vi "Control - Diesel - Cranking.vi"(0 "Control Inputs":T4={"Engine Speed [RPM]"=0.0, "Engine Status"=enum."STALLED", "Load Control \nMode"=enum."High-Idle Governor", "dt(s)"=0.0, "Number of Cylinders"=0, "Engine Displacement [cc]"=0.0, "StoichAFR"=0.0, "Q.LHV Fuel [kJ/kg]"=0.0, "BattV PSU [V]"=0.0, "12V PSU [V]"=0.0, "5V PSU [V]"=0.0, "Pedal Position [%]"=0.0, "Oil Pressure [kPa]"=0.0, "Oil Temp [C]"=0.0, "Oil Level [%]"=0.0, "Engine Coolant Temp (ECT) [C]"=0.0, "Engine Coolant Pressure [kPa]"=0.0, "Rail Pressure [bar]"=0.0, "Fuel Pressure [kPa]"=0.0, "Fuel Temp [C]"=0.0, "Vacuum Pressure [kPa]"=0.0, "Throttle Position [%]"=0.0, "Cam1 Advance [CAD]"=0.0, "Cam2 Advance [CAD]"=0.0, "Cam3 Advance [CAD]"=0.0, "Cam4 Advance [CAD]"=0.0, "CA50 Control Output [CAD]"=[], "CA50 Control Output Valid"=[], "Intake Air Temp (IAT) [C]"=0.0, "Barometric Air Pressure [kPa]"=0.0, "Intake Air Rel. Humidity [%]"=0.0, "Mass Air Flow (MAF) [kg/hr]"=0.0, "Turbo Inlet Air Pressure [kPa]"=0.0, "Turbo Inlet Air Temp [C]"=0.0, "Turbo Outlet Air Pressure [kPa]"=0.0, "Turbo Outlet Air Temp [C]"=0.0, "CAC Outlet Pressure [kPa]"=0.0, "CAC Outlet Temp [C]"=0.0, "Intake Manifold Pressure (MAP) [kPa]"=0.0, "Intake Manifold Temp (MAT) [C]"=0.0, "Exhaust Manifold Pressure [kPa]"=0.0, "Exhaust Manifold Temp [C]"=0.0, "HighP EGR Cooler Outlet Pressure [kPa]"=0.0, "HighP EGR Cooler Outlet Temp [C]"=0.0, "HighP EGR Differential Pressure [kPa]"=0.0, "HighP EGR Valve Position [%]"=0.0, "Turbo Outlet Exhaust Pressure [kPa]"=0.0, "Turbo Outlet Exhaust Temp [C]"=0.0, "VGT Position 1 [%]"=0.0, "VGT Position 2 [%]"=0.0, "Turbo Speed 1 [RPM]"=0.0, "Turbo Speed 2 [RPM]"=0.0, "LowP EGR Differential Pressure [kPa]"=0.0, "LowP EGR Valve Position [%]"=0.0, "UEGO1Lambda"=0.0, "UEGO1_Hot"=FALSE, "UEGO2Lambda"=0.0, "UEGO2_Hot"=FALSE, "Knock Intensity"=[], "Knock"=[]} {"Knock Intensity" format="%.2f"; "CA50 Control Output [CAD]" format="%.2f"; "Exhaust Manifold Temp [C]" format="%#_6f"; "UEGO2Lambda" format="%.2f"; "Intake Manifold Temp (MAT) [C]" format="%#_6f"; "UEGO1Lambda" format="%.2f"}, 1 "Available Air Mass [mg/cyc]":sgl, 5 "Control Outputs In":T1) -> (19 "Control Outputs":T1)   [LabVIEW 2015, in "ECS-RT.lvlib"]
uses:
  ECS-RT.lvlib
  Typedefs/Control Inputs/Control Inputs.ctl
  Typedefs/EPT/Engine Status.ctl
  Typedefs/MISC/Load Control Mode.ctl
  Typedefs/Control Outputs/Control Outputs.ctl
  Typedefs/Control Outputs/Injection Quantity.ctl
  Typedefs/Control Outputs/Injection Timing.ctl
  ECS-Shared.lvlib
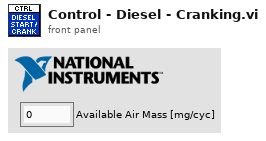
[diagram p1: front panel]
types:
  T1 = typedef "ECS-Shared.lvlib/Control Outputs.ctl" = cluster{"Pedal Desired [%]":sgl, "MEP Desired [bar]":sgl, "Fuel Desired [mg/cyc]":sgl, "Intake MAP Desired [kPa]":sgl, "Cam1 Advance Setpoint [CAD]":sgl, "Cam2 Advance Setpoint [CAD]":sgl, "HighP EGR Position Setpoint [%Open]":sgl, "LowP EGR Position Setpoint [%Open]":sgl, "Rail Pressure Setpoint [bar]":sgl, "Wastegate1 Position Setpoint [%Open]":sgl, "Wastegate2 Position Setpoint [%Open]":sgl, "VGT1 Position Setpoint [%Open]":sgl, "VGT2 Position Setpoint [%Open]":sgl, "Throttle1 Position Setpoint [%Open]":sgl, "Throttle2 Position Setpoint [%Open]":sgl, "TurboBPV Position Setpoint [%Open]":sgl, "Spark Dwells [msec]":sgl[], "Spark Timings [DBTDC]":sgl[], "PFI Quantities [mg/inj]":sgl[], "PFI Timings [DBTDC]":sgl[], "DI Quantities [mg/inj]":T2[], "DI Timings [DBTDC]":T3[]}
  T2 = typedef "ECS-Shared.lvlib/Injection Quantity.ctl" = cluster{"Pilot1Quantity [mg/inj]":sgl, "Pilot2Quantity [mg/inj]":sgl, "MainQuantity [mg/inj]":sgl, "Post1Quantity [mg/inj]":sgl, "Post2Quantity [mg/inj]":sgl}
  T3 = typedef "ECS-Shared.lvlib/Injection Timing.ctl" = cluster{"Pilot1SOI [DBTDC]":sgl, "Pilot2SOI [DBTDC]":sgl, "MainSOI [DBTDC]":sgl, "Post1SOI [DBTDC]":sgl, "Post2SOI [DBTDC]":sgl}
  T4 = typedef "ECS-Shared.lvlib/Control Inputs.ctl" = cluster{"Engine Speed [RPM]":sgl, "Engine Status":T5, "Load Control \nMode":T6, "dt(s)":sgl, "Number of Cylinders":u8, "Engine Displacement [cc]":sgl, "StoichAFR":sgl, "Q.LHV Fuel [kJ/kg]":sgl, "BattV PSU [V]":sgl, "12V PSU [V]":sgl, "5V PSU [V]":sgl, "Pedal Position [%]":sgl, "Oil Pressure [kPa]":sgl, "Oil Temp [C]":sgl, "Oil Level [%]":sgl, "Engine Coolant Temp (ECT) [C]":sgl, "Engine Coolant Pressure [kPa]":sgl, "Rail Pressure [bar]":sgl, "Fuel Pressure [kPa]":sgl, "Fuel Temp [C]":sgl, "Vacuum Pressure [kPa]":sgl, "Throttle Position [%]":sgl, "Cam1 Advance [CAD]":sgl, "Cam2 Advance [CAD]":sgl, "Cam3 Advance [CAD]":sgl, "Cam4 Advance [CAD]":sgl, "CA50 Control Output [CAD]":sgl[], "CA50 Control Output Valid":bool[], "Intake Air Temp (IAT) [C]":sgl, "Barometric Air Pressure [kPa]":sgl, "Intake Air Rel. Humidity [%]":sgl, "Mass Air Flow (MAF) [kg/hr]":sgl, "Turbo Inlet Air Pressure [kPa]":sgl, "Turbo Inlet Air Temp [C]":sgl, "Turbo Outlet Air Pressure [kPa]":sgl, "Turbo Outlet Air Temp [C]":sgl, "CAC Outlet Pressure [kPa]":sgl, "CAC Outlet Temp [C]":sgl, "Intake Manifold Pressure (MAP) [kPa]":sgl, "Intake Manifold Temp (MAT) [C]":sgl, "Exhaust Manifold Pressure [kPa]":sgl, "Exhaust Manifold Temp [C]":sgl, "HighP EGR Cooler Outlet Pressure [kPa]":sgl, "HighP EGR Cooler Outlet Temp [C]":sgl, "HighP EGR Differential Pressure [kPa]":sgl, "HighP EGR Valve Position [%]":sgl, "Turbo Outlet Exhaust Pressure [kPa]":sgl, "Turbo Outlet Exhaust Temp [C]":sgl, "VGT Position 1 [%]":sgl, "VGT Position 2 [%]":sgl, "Turbo Speed 1 [RPM]":sgl, "Turbo Speed 2 [RPM]":sgl, "LowP EGR Differential Pressure [kPa]":sgl, "LowP EGR Valve Position [%]":sgl, "UEGO1Lambda":sgl, "UEGO1_Hot":bool, "UEGO2Lambda":sgl, "UEGO2_Hot":bool, "Knock Intensity":sgl[], "Knock":bool[]}
  T5 = typedef "ECS-Shared.lvlib/Engine Status.ctl" = enum16{"OFF", "STALLED", "CRANKING", "RUNNING", "ACCEL", "DECEL", "SAFE"}
  T6 = typedef "ECS-Shared.lvlib/Load Control Mode.ctl" = enum16{"No Governor", "Low-Idle Governor", "High-Idle Governor"}
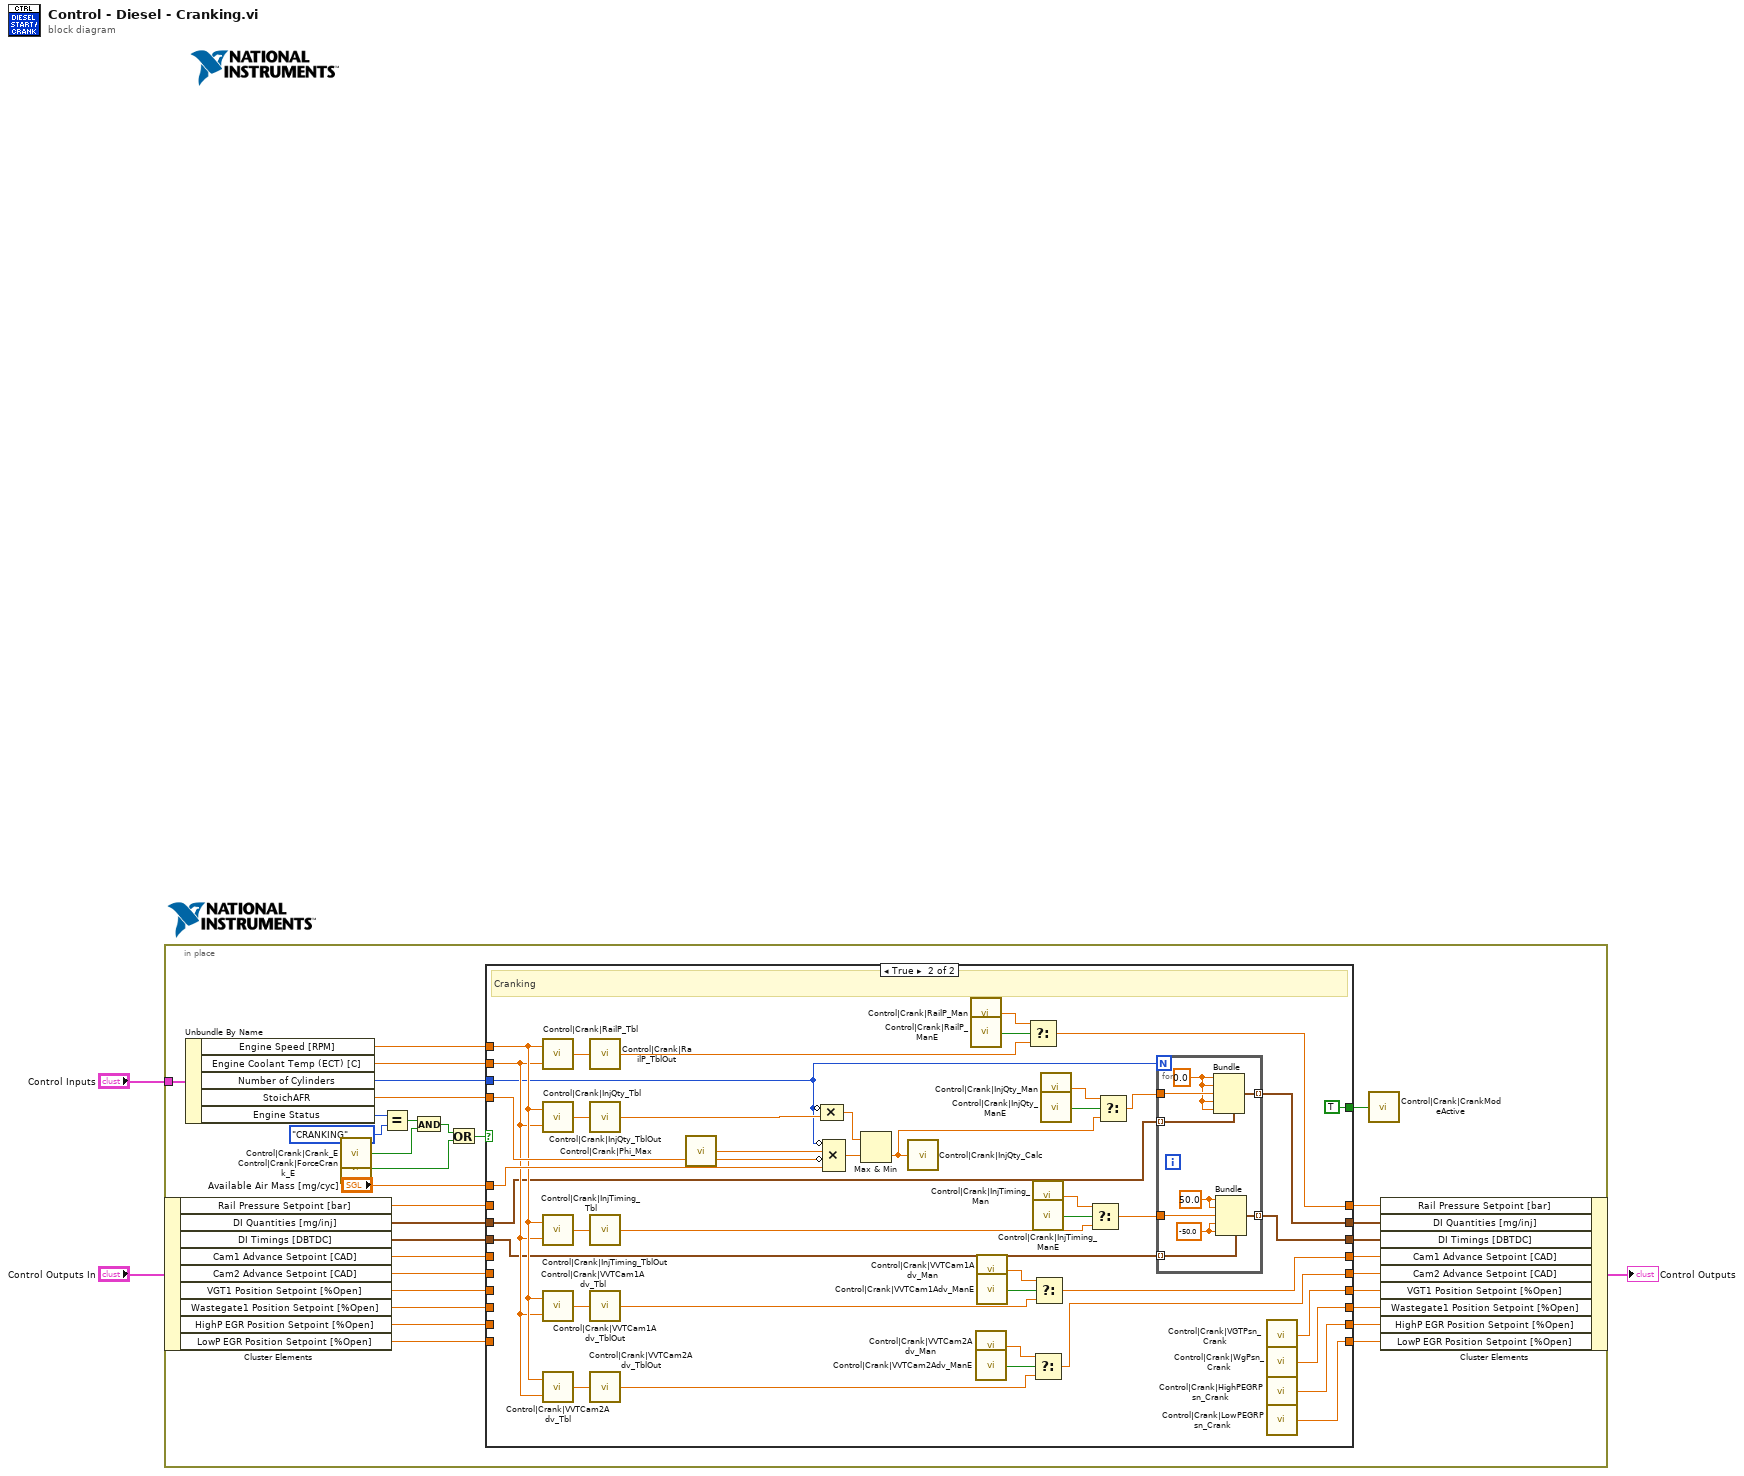
[diagram p0: block diagram]
diagram:
  n1 = in-place {
    in-place-border: "Control Inputs" -> [w31]
    n2 = in-place-cluster #1("Control Outputs In") -> ("Rail Pressure Setpoint [bar]"=w21:sgl, "DI Quantities [mg/inj]"=w20:T2[], "DI Timings [DBTDC]"=w19:T3[], "Cam1 Advance Setpoint [CAD]"=w18:sgl, "Cam2 Advance Setpoint [CAD]"=w17:sgl, "VGT1 Position Setpoint [%Open]"=w16:sgl, "Wastegate1 Position Setpoint [%Open]"=w15:sgl, "HighP EGR Position Setpoint [%Open]"=w14:sgl, "LowP EGR Position Setpoint [%Open]"=w13:sgl)
    n3 = Unbundle By Name(w31) -> ("Engine Speed [RPM]"=w35:sgl, "Engine Coolant Temp (ECT) [C]"=w34:sgl, "Number of Cylinders"=w33:u8, "StoichAFR"=w32:sgl, "Engine Status"=w29:T5)
    n4 = call "Control|Crank|Crank_E"() -> ("Value"=w26:bool)
    n5 = call "Control|Crank|ForceCrank_E"() -> ("Value"=w24:bool)
    n6 = Equal?(x=w29, y=Engine_Status."CRANKING" ("Engine Status")) -> (x = y?=w27:bool)
    n7 = And(x=w27, y=w26) -> (x .and. y?=w23:bool)
    n8 = Or(x=w23, y=w24) -> (x .or. y?=w25:bool)
    n9 = case shown="True" w25 {
      tunnel: w35 -> [_ w59]
      tunnel: w34 -> [_ w58]
      tunnel: w33 -> [_ w45]
      tunnel: w32 -> [_ w73]
      tunnel: "Available Air Mass [mg/cyc]" -> [_ w72]
      tunnel: [_ TRUE] -> w30
      tunnel: w21 -> [w36 _]
      tunnel: w20 -> [w37 w51]
      tunnel: w19 -> [w38 w46]
      tunnel: w18 -> [w39 _]
      tunnel: w17 -> [w40 _]
      tunnel: w16 -> [w41 _]
      tunnel: w15 -> [w42 _]
      tunnel: w14 -> [w43 _]
      tunnel: w13 -> [w44 _]
      tunnel: [w44 w52] -> w12
      tunnel: [w43 w53] -> w11
      tunnel: [w42 w54] -> w10
      tunnel: [w41 w55] -> w9
      tunnel: [w40 w56] -> w8
      tunnel: [w39 w57] -> w7
      tunnel: [w38 w47] -> w6
      tunnel: [w37 w49] -> w5
      tunnel: [w36 w78] -> w4
      frame False {
        # "Normal Operation"
      }
      frame True {
        # "Cranking"
        n10 = call "Control|Crank|RailP_Tbl"("Y Index"=w58, "X Index"=w59) -> ("Z"=w81:sgl)
        n11 = call "Control|Crank|InjQty_Tbl"("Y Index"=w58, "X Index"=w59) -> ("Z"=w74:sgl)
        n12 = call "Control|Crank|InjTiming_Tbl"("Y Index"=w58, "X Index"=w59) -> ("Z"=w68:sgl)
        n13 = call "Control|Crank|VVTCam1Adv_Tbl"("Y Index"=w58, "X Index"=w59) -> ("Z"=w62:sgl)
        n14 = call "Control|Crank|VVTCam2Adv_Tbl"("Y Index"=w58, "X Index"=w59) -> ("Z"=w63:sgl)
        n15 = call "Control|Crank|RailP_TblOut"("Value"=w81) -> ()
        n16 = call "Control|Crank|InjQty_TblOut"("Value"=w74) -> ()
        n17 = call "Control|Crank|InjTiming_TblOut"("Value"=w68) -> ()
        n18 = call "Control|Crank|VVTCam1Adv_TblOut"("Value"=w62) -> ()
        n19 = call "Control|Crank|VVTCam2Adv_TblOut"("Value"=w63) -> ()
        n20 = call "Control|Crank|Phi_Max"() -> ("Value"=w75:sgl)
        n21 = Compound Arithmetic op=MULTIPLY(invert w45, w74) -> (w76:dbl)
        n22 = Compound Arithmetic op=MULTIPLY(invert w45, w75, invert w73, w72) -> (w77:dbl)
        n23 = Max & Min(x=w76, y=w77) -> (min(x,y)=w69:dbl)  [unwired: 1 out]
        n24 = call "Control|Crank|InjQty_Calc"("Value"=w69) -> ()
        n25 = call "Control|Crank|RailP_Man"() -> ("Value"=w79:sgl)
        n26 = call "Control|Crank|RailP_ManE"() -> ("Value"=w80:bool)
        n27 = call "Control|Crank|VVTCam2Adv_Man"() -> ("Value"=w65:sgl)
        n28 = call "Control|Crank|VVTCam2Adv_ManE"() -> ("Value"=w64:bool)
        n29 = call "Control|Crank|VVTCam1Adv_Man"() -> ("Value"=w60:sgl)
        n30 = call "Control|Crank|VVTCam1Adv_ManE"() -> ("Value"=w61:bool)
        n31 = Select(t=w79, s=w80, f=w81) -> (s? t:f=w78:sgl)
        n32 = call "Control|Crank|InjTiming_Man"() -> ("Value"=w67:sgl)
        n33 = call "Control|Crank|InjTiming_ManE"() -> ("Value"=w66:bool)
        n34 = Select(t=w65, s=w64, f=w63) -> (s? t:f=w56:sgl)
        n35 = Select(t=w60, s=w61, f=w62) -> (s? t:f=w57:sgl)
        n36 = call "Control|Crank|InjQty_Man"() -> ("Value"=w71:sgl)
        n37 = call "Control|Crank|InjQty_ManE"() -> ("Value"=w70:bool)
        n38 = Select(t=w67, s=w66, f=w68) -> (s? t:f=w48:sgl)
        n39 = Select(t=w71, s=w70, f=w69) -> (s? t:f=w50:dbl)
        n40 = for {
          N: w45 -> [_]
          tunnel: [w91] -> w49 mode=indexing
          tunnel: w51 -> [w90] mode=indexing
          tunnel: w50 -> [w89]
          tunnel: w48 -> [w85]
          tunnel: [w84] -> w47 mode=indexing
          tunnel: w46 -> [w83] mode=indexing
          w87 = sgl -50.0 ("Pilot1SOI [DBTDC]")
          w86 = sgl 50.0 ("Pilot1SOI [DBTDC]")
          w88 = sgl 0.0 ("Pilot1Quantity [mg/inj]")
          n41 = Bundle(cluster=w90, "Pilot1Quantity [mg/inj]"=w88, "Pilot2Quantity [mg/inj]"=w88, "MainQuantity [mg/inj]"=w89, "Post1Quantity [mg/inj]"=w88, "Post2Quantity [mg/inj]"=w88) -> (w91:T2)
          n42 = Bundle(cluster=w83, "Pilot1SOI [DBTDC]"=w86, "Pilot2SOI [DBTDC]"=w86, "MainSOI [DBTDC]"=w85, "Post1SOI [DBTDC]"=w87, "Post2SOI [DBTDC]"=w87) -> (w84:T3)
        }
        n43 = call "Control|Crank|VGTPsn_Crank"() -> ("Value"=w55:sgl)
        n44 = call "Control|Crank|WgPsn_Crank"() -> ("Value"=w54:sgl)
        n45 = call "Control|Crank|HighPEGRPsn_Crank"() -> ("Value"=w53:sgl)
        n46 = call "Control|Crank|LowPEGRPsn_Crank"() -> ("Value"=w52:sgl)
      }
    }
    n47 = call "Control|Crank|CrankModeActive"("Value"=w30) -> ()
    n48 = in-place-cluster #1("Rail Pressure Setpoint [bar]"=w4, "DI Quantities [mg/inj]"=w5, "DI Timings [DBTDC]"=w6, "Cam1 Advance Setpoint [CAD]"=w7, "Cam2 Advance Setpoint [CAD]"=w8, "VGT1 Position Setpoint [%Open]"=w9, "Wastegate1 Position Setpoint [%Open]"=w10, "HighP EGR Position Setpoint [%Open]"=w11, "LowP EGR Position Setpoint [%Open]"=w12) -> (→"Control Outputs":T1)
  }
